vi "Configure Analog Input Sensor.vi"(0 "VISA resource name":refnum<visa-resource-name>, 1 "Analog Input (1)":i16=1, 2 "Altitude (0: 0 to 2499 ft)":i16(ring) items=["0 to 2499 ft", "2500 to 4999 ft", "5000 ft and above"], 3 "Units (0: Temperature)":u16(ring) items=["Temperature", "% rh", "Psi", "Units"], 4 "Decimal Point (0: 0)":u16(ring) items=["0", "0.0", "0.00 process", "0.000 process"], 5 "error in (no error)":errorcluster {"code" format="%.0x"}, 6 "Unit Address (1)":i16=1, 8 "Sensor (0: Thermocouple)":u16(ring) items=["Thermocouple", "RTD", "Process", "Wet Bulb - Dry Bulb", "Off"], 10 "Type (0: J)":u16(ring) items=["J", "K", "T", "E", "N", "C", "D", "PT2", "R", "S", "B", "100 ohm DIN", "100 ohm JIS", "4 to 20 mA", "0 to 20 mA", "0 to 5 V", "1 to 5 V", "0 to 10 V", "0 to 50 mV", "Vaisala 0 to 5 V", "Vaisala 0 to 10 V", "Vaisala 0 to 20 mA", "Rotronics 0 to 5 V", "500 ohm DIN", "500 ohm JIS", "1000 ohm DIN", "1000 ohm JIS"]) -> (14 "VISA resource name out":refnum<visa-resource-name>, 19 "error out":errorcluster {"code" format="%.0x"})   [LabVIEW 2010]
doc: "This VI is used to configure analog inputs.\n\nCaution:\nAll profiles stored in the WLF4's memory will be deleted.\n\nNote:\nThe last two digits of your model number determines your RTD base resistance:\nF4XX-XXXX-XXRG - 100 ohms\nF4XX-XXXX-XXRH - 500 ohms and 1 kohm"
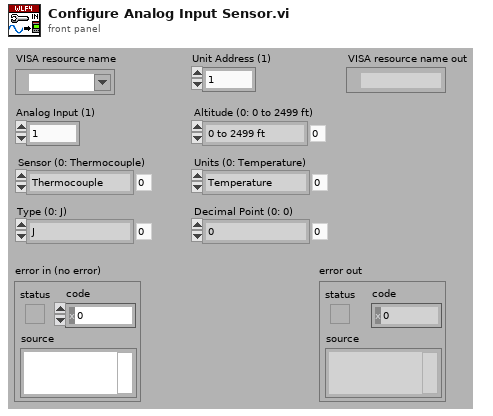
[diagram p1: front panel]
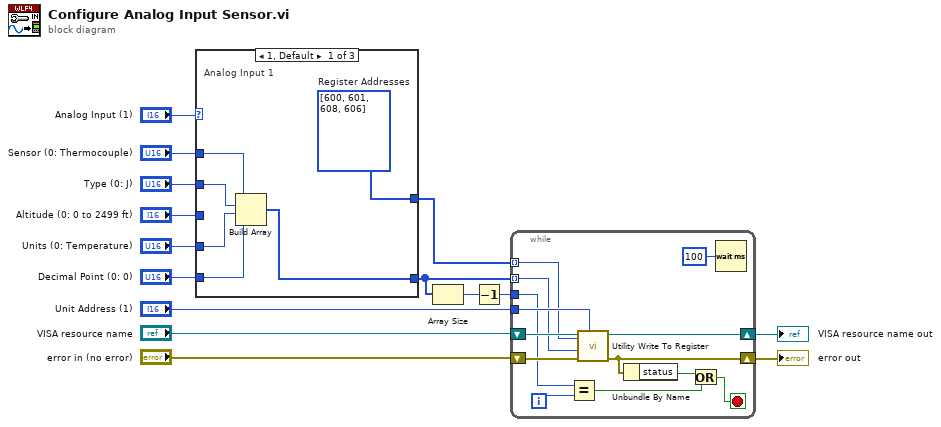
[diagram p0: block diagram]
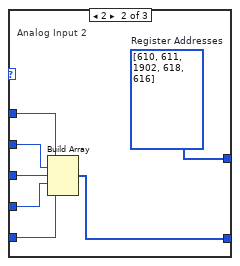
[diagram p2: hidden frame]
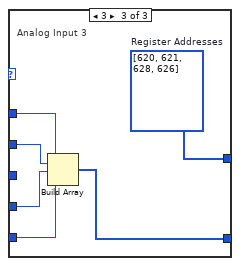
[diagram p3: hidden frame]
diagram:
  n1 = case shown="1, Default" "Analog Input (1)" {
    tunnel: [w21 w28 w34] -> w10
    tunnel: "Sensor (0: Thermocouple)" -> [w20 w26 w33]
    tunnel: "Type (0: J)" -> [w18 w25 w32]
    tunnel: "Units (0: Temperature)" -> [w17 w23 w31]
    tunnel: "Decimal Point (0: 0)" -> [w19 w27 w30]
    tunnel: [w16 w22 w29] -> w3
    tunnel: "Altitude (0: 0 to 2499 ft)" -> [_ w24 _]
    frame 1, Default {
      w21 = i32[] [600, 601, 608, 606]  # Register Addresses
      # "Analog Input 1"
      n2 = Build Array(w20, w18, w17, w19) -> (w16:u16[])
    }
    frame 2 {
      w28 = i32[] [610, 611, 1902, 618, 616]  # Register Addresses
      # "Analog Input 2"
      n3 = Build Array(w26, w25, w24, w23, w27) -> (w22:u16[])
    }
    frame 3 {
      w34 = i32[] [620, 621, 628, 626]  # Register Addresses
      # "Analog Input 3"
      n4 = Build Array(w33, w32, w31, w30) -> (w29:u16[])
    }
  }
  n5 = Array Size(array=w3) -> (size(s)=w2:i32)
  n6 = Decrement(x=w2) -> (x-1=w1:i32)
  n7 = while {
    tunnel: "Unit Address (1)" -> [w47]
    shift-right: [w44] -> w13
    shift-left: "VISA resource name" -> [w46]
    shift-right: [w41] -> w12
    shift-left: "error in (no error)" -> [w45]
    tunnel: w10 -> [w42] mode=indexing
    tunnel: w3 -> [w36] mode=indexing
    tunnel: w1 -> [w35]
    i -> [w38]
    stop <- w40 stop-if-true
    n8 = Equal?(x=w35, y=w38) -> (x = y?=w37:bool)
    n9 = call "Utility Write To Register.vi"("Unit Address (1)"=w47, "error in (no error)"=w45, "Data (0)"=w36, "Register Address (0)"=w42, "VISA resource name"=w46) -> ("error out"=w41:errorcluster, "VISA resource name out"=w44:refnum<visa-resource-name>)  [unwired: 5 in]
    n10 = Unbundle By Name(w41) -> ("status"=w39:bool)
    n11 = Or(x=w39, y=w37) -> (x .or. y?=w40:bool)
    n12 = Wait (ms)(milliseconds to wait=u32 100) -> ()  [unwired: 1 out]
  }
  "error out" <- w12
  "VISA resource name out" <- w13
